vi "_script_fix_list event frames.vi"   [LabVIEW 2014]
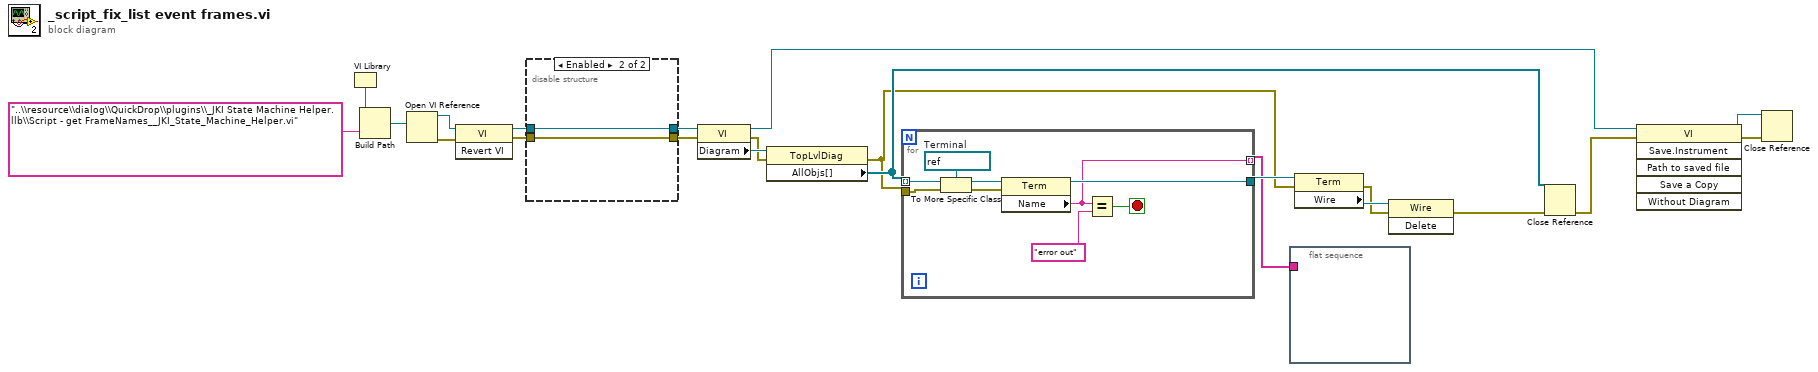
[diagram p0: block diagram]
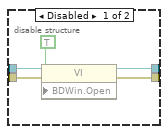
[diagram p2: hidden frame]
diagram:
  n1 = VI Library() -> (path=w20:path)
  n2 = Build Path(base path=w20, name or relative path="..\\resource\\dialog\\QuickDrop\\plugins\\_JKI State Machine Helper.llb\\Script - get FrameNames__JKI_State_Machine_Helper.vi") -> (appended path=w18:path)
  n3 = Open VI Reference(vi path=w18) -> (vi reference=w21:refnum<vi>, error out=w22:errorcluster)  [unwired: 5 in]
  n4 = invoke class="VI" method="Revert VI"(reference=w21, error in=w22) -> (reference out=w15:refnum<vi>, error out=w14:errorcluster)  [unwired: 1 in, 1 out]
  n5 = disable-structure shown="Enabled" {
    disable-tunnel: w15 -> [w27 w29]
    disable-tunnel: w14 -> [w26 w28]
    disable-tunnel: [w25 w29] -> w13
    disable-tunnel: [w24 w28] -> w12
    frame Disabled {
      n6 = property class="VI"(reference=w27, error in=w26, "BDWin.Open"=TRUE ("Block Diagram Window:Open")) -> (reference out=w25:refnum<vi>, error out=w24:errorcluster)
    }
    frame Enabled {
    }
  }
  n7 = property class="VI"(reference=w13, error in=w12) -> (reference out=w6:refnum<vi>, error out=w10:errorcluster, "Diagram"=w11:refnum<vi>)
  n8 = property class="TopLvlDiag"(reference=w11, error in=w10) -> (error out=w2:errorcluster, "AllObjs[]"=w4:refnum<vi>[])  [unwired: 1 out]
  n9 = for {
    tunnel: w4 -> [w38] mode=indexing
    tunnel: [w33] -> w9
    tunnel: w2 -> [w32]
    tunnel: [w30] -> w1 mode=indexing
    stop <- w34 stop-if-true
    w36 = refnum<vi> refnum  # Terminal
    n10 = To More Specific Class(target class=w36, reference=w38, error in=w32) -> (specific class reference=w37:refnum<vi>, error out=w31:errorcluster)
    n11 = property class="Term"(reference=w37, error in=w31) -> (reference out=w33:refnum<vi>, "Name"=w30:string)  [unwired: 1 out]
    n12 = Equal?(x=w30, y="error out") -> (x = y?=w34:bool)
  }
  n13 = flat-sequence {
    tunnel: w1 -> [_]
    frame #0 {
    }
  }
  n14 = property class="Term"(reference=w9, error in=w2) -> (error out=w7:errorcluster, "Wire"=w8:refnum<vi>)  [unwired: 1 out]
  n15 = invoke class="Wire" method="Delete"(reference=w8, error in=w7) -> (error out=w3:errorcluster)  [unwired: 1 in, 2 out]
  n16 = Close Reference(reference=w4, error in (no error)=w3) -> (error out=w5:errorcluster)
  n17 = invoke class="VI" method="Save.Instrument"(reference=w6, error in=w5) -> (reference out=w16:refnum<vi>, error out=w17:errorcluster)  [unwired: 4 in, 4 out]
  n18 = Close Reference(reference=w16, error in (no error)=w17) -> ()  [unwired: 1 out]
